vi "oea.vi"() -> ()   [LabVIEW 2013]
uses:
  <vilib>/Analysis/NI_AALPro.lvlib
  <vilib>/robotics/Kinematics/NI_Kinematics.lvlib
panel:
  out "Cross Product":dbl[](array[numeric])
  in  "a":dbl[](array[numeric])=[1.0, 1.0, 1.0, 1.0]
  in  "o":dbl[](array[numeric])=[1.0, 1.0, 1.0, 1.0]
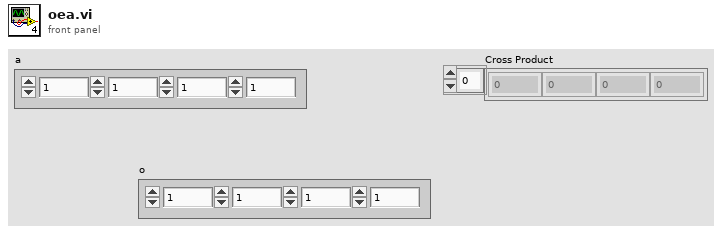
[diagram p1: front panel]
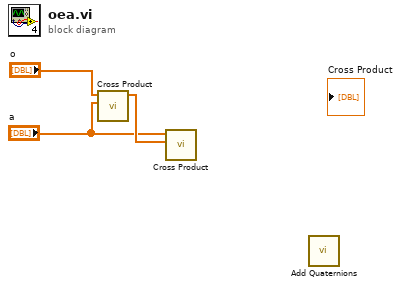
[diagram p0: block diagram]
diagram:
  n1 = call <vilib>:"Cross Product.vi"("B Vector"="a", "A Vector"="o") -> ("Cross Product"=w2:dbl[])  [unwired: 8 in, 1 out]
  n2 = call <vilib>:"Cross Product.vi"("B Vector"=w2, "A Vector"="a") -> ()  [unwired: 8 in, 2 out]
  n3 = call <vilib>:"Add Quaternions.vi"() -> ()  [unwired: 2 in, 1 out]
